vi "제목없음 4.vi"() -> ()   [LabVIEW 2019]
uses:
  Users/Wego/Documents/GitHub/ERP42-v2/Ctrl/clamp-result_cmd.ctl
  <vilib>/Analysis/baseanly.llb/Mean (DBL).vi
  <vilib>/Analysis/NI_AALBase.lvlib
panel:
  out "웨이브폼 차트":cluster{"x-center":dbl, "mean":dbl}(graph)
  in  "정지":bool
  out "XY 그래프 2":cluster{"X":sgl, "Y":sgl}[](graph)
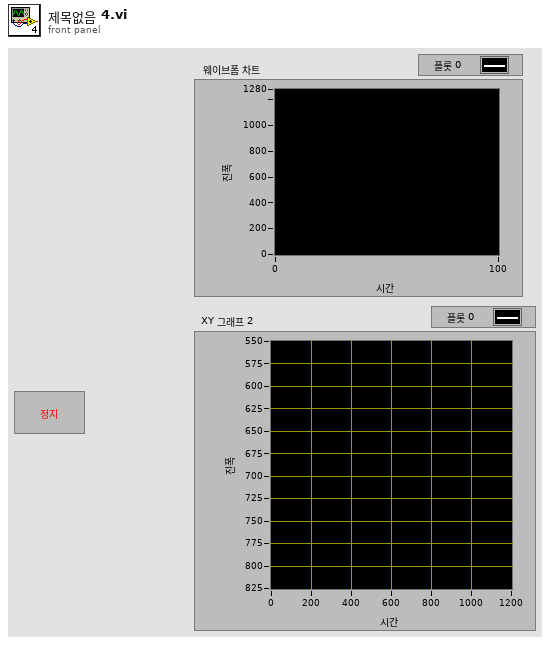
[diagram p1: front panel]
types:
  T1 = typedef "clamp-result_cmd.ctl" = enum16{"write_clamp_overlay-result", "write_center-distance", "write_clamp_result", "write_threshold_result", "read"}
  T2 = typedef "ROI Descriptor" = cluster{"Global Rectangle":i32[], "Contours":cluster{"ID":enum32{"External", "Internal"}, "Type":u32, "Coordinates":i32[]}[]}
  T3 = cluster{"Points":cluster{"X":sgl, "Y":sgl}[], "Points2":cluster{"X":sgl, "Y":sgl}[], "Point3":cluster{cluster{"X":sgl, "Y":sgl}, cluster{"X":sgl, "Y":sgl}}[], "Perpendicular Lines":cluster{cluster{"X":sgl, "Y":sgl}, cluster{"X":sgl, "Y":sgl}}[], "ROI Descriptor out":T2}
  T4 = cluster{"x-center":dbl, "Image Size":cluster{"x":i32, "y":i32}, "Angle deg":sgl, "Threshold Range":cluster{"Lower value":sgl, "Upper value":sgl}}
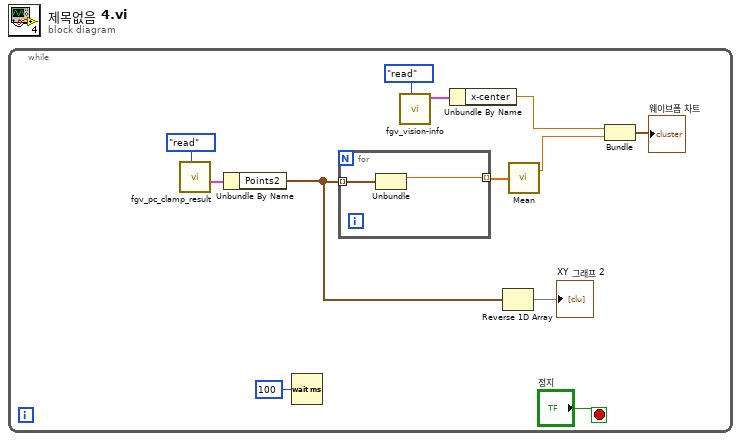
[diagram p0: block diagram]
diagram:
  n1 = while {
    stop <- "정지" stop-if-true
    n2 = call "fgv_pc_clamp_result.vi"("cmd"=clamp-result_cmd."read") -> ("clamp_roi_overlay-result_out"=w11:T3)  [unwired: 7 in, 3 out]
    n3 = Unbundle By Name(w11) -> ("Points2"=w1:cluster{"X":sgl, "Y":sgl}[])
    n4 = Wait (ms)(milliseconds to wait=u32 100 ("대기 시간 (ms)")) -> ()  [unwired: 1 out]
    n5 = for {
      tunnel: w1 -> [w14] mode=indexing
      tunnel: [w13] -> w7 mode=indexing
      n6 = Unbundle(w14) -> ("X"=w13:sgl)  [unwired: 1 out]
    }
    n7 = call "fgv_vision-info.vi"("cmd"=enum16{"read", "write"}."read") -> ("image info out"=w5:T4)  [unwired: 10 in]
    n8 = Unbundle By Name(w5) -> ("x-center"=w3:dbl)
    n9 = Reverse 1D Array(array=w1) -> (reversed array=→"XY 그래프 2":cluster{"X":sgl, "Y":sgl}[])
    n10 = call-poly <vilib>:"Mean.vi"("X"=w7) -> ("mean"=w4:dbl)  [unwired: 1 out]
    n11 = Bundle("x-center"=w3, "mean"=w4) -> (→"웨이브폼 차트":cluster{"x-center":dbl, "mean":dbl})  [unwired: 1 in]
  }
